vi "GraphSetup.vi"(8 "error in":errorcluster caption="entrée d'erreur (pas d'erreur)", 9 "AllowDef":bool, 10 "DataFileName":path, 11 "InterfaceIn":refnum<class "Interface.lvclass">) -> (0 "error out":errorcluster caption="sortie d'erreur", 3 "InterfaceOut":refnum<class "Interface.lvclass">)   [LabVIEW 2019, in "Interface.lvclass"]
uses:
  Interface.lvclass
  GraphSetupStates.ctl
  Interface.lvclass/Interface.ctl
  <vilib>/Utility/error.llb/DialogType.ctl
panel:
  out "DataIndex":i32[](array[numeric])
  out "DataCount":i32
  out "ScanlistItem":string
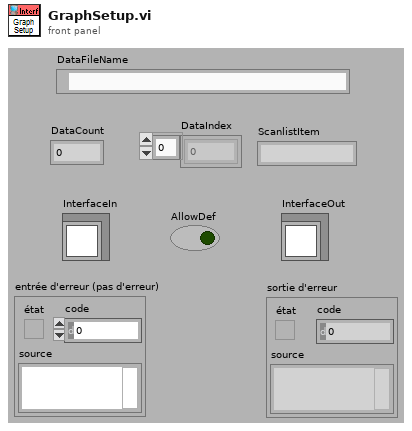
[diagram p1: front panel]
types:
  T1 = typedef "Interface.lvclass/GraphSetupStates.ctl" = enum16{"RdScnList", "UpdtGrphCurvs", "UpdtAllCurv", "SetGraphPar", "UpdtCrvPar", "GetNextItem", "UpdateGraph"}
  T2 = typedef "Interface.lvclass/CurveSetup.ctl" = cluster{"CurveName":string, "YParam":string, "XParam":string, "ZParam ":string, "GroupName":string, "LinWdth":u8, "PntCol":u32, "LinCol":u32, "LablFor":u8, "XScale":u32, "YScale":u32, "Interpol":u8, "DisplayName":string, "FillType":i16, "LineStyle":u8, "PntStyle":u8, "BarTyp":u8, "GraphIndex":i32, "Visible":bool, "XScaleName":string, "YScaleName":string, "XYGraph_Ref":refnum<vi>, "Data Only":bool, "DataQ Ref":refnum<queue>, "XParQ Ref":refnum<queue>, "XParamInd":i32, "ScanInd":i32, "File Path":path}
  T3 = typedef "DialogType.ctl" = u16
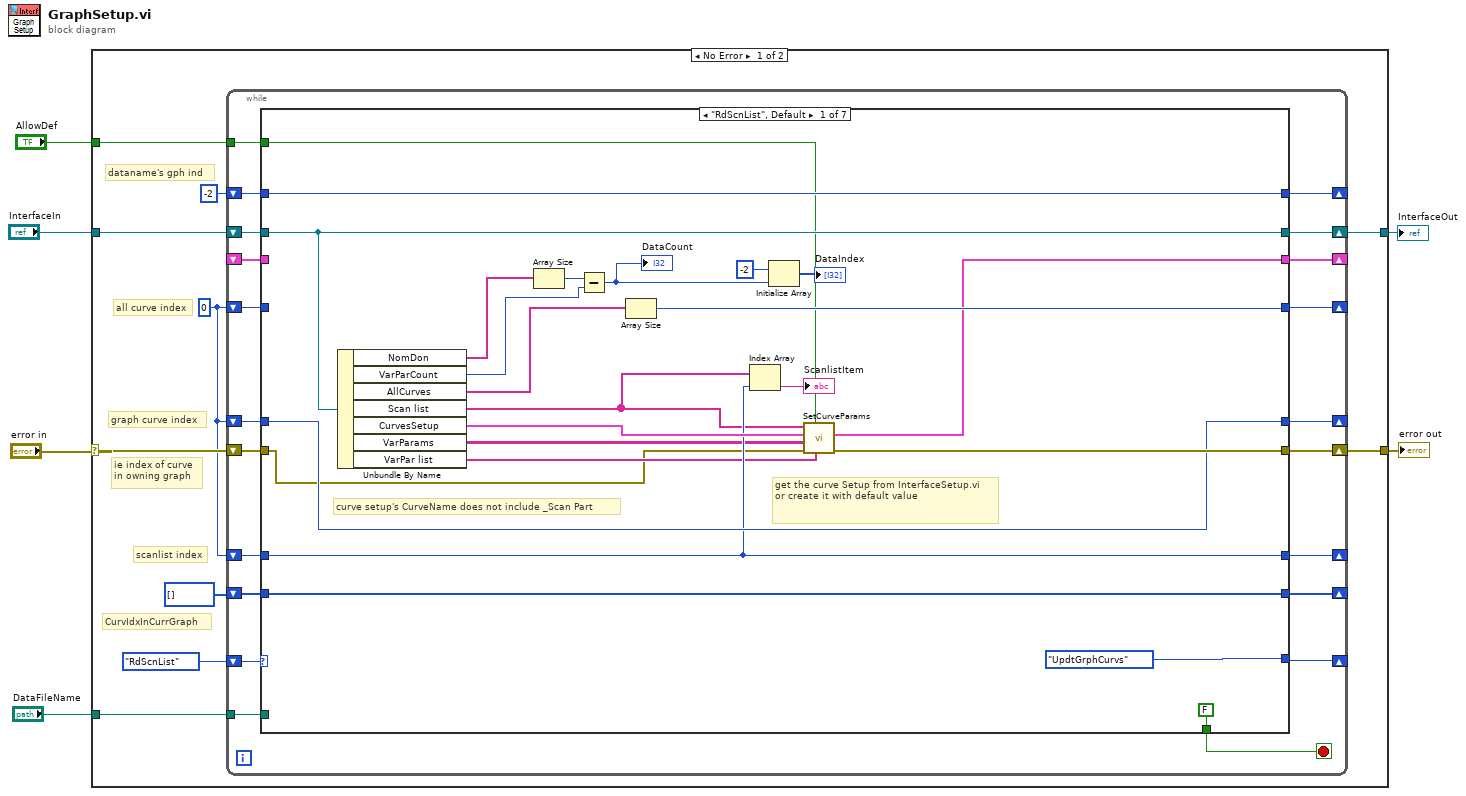
[diagram p0: block diagram]
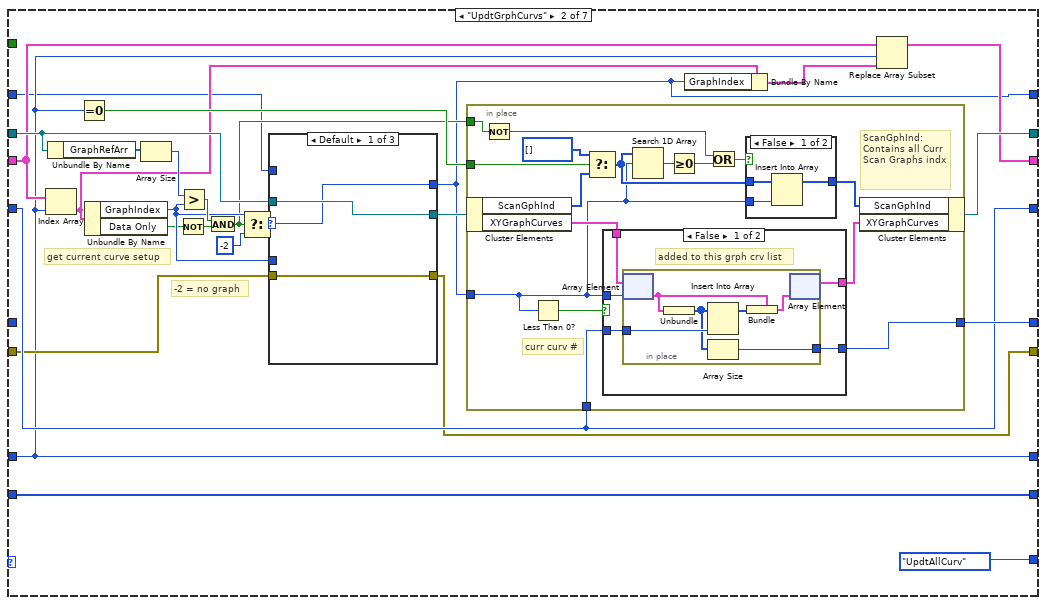
[diagram p2: hidden frame]
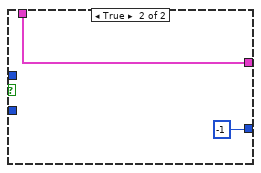
[diagram p3: hidden frame]
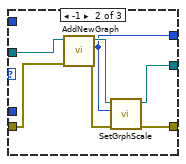
[diagram p5: hidden frame]
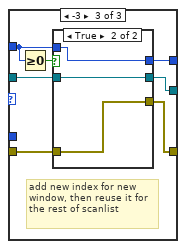
[diagram p6: hidden frame]
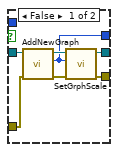
[diagram p7: hidden frame]
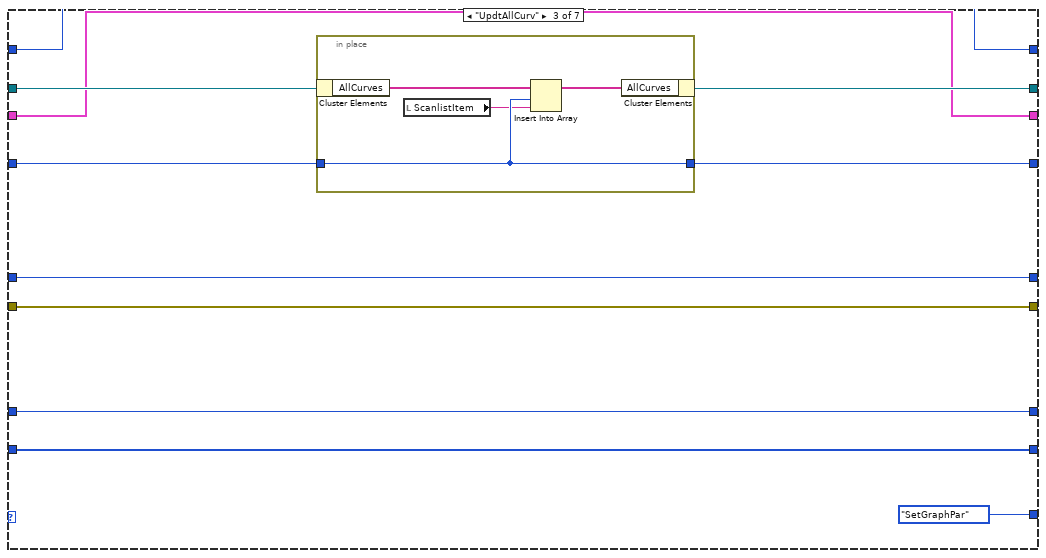
[diagram p8: hidden frame]
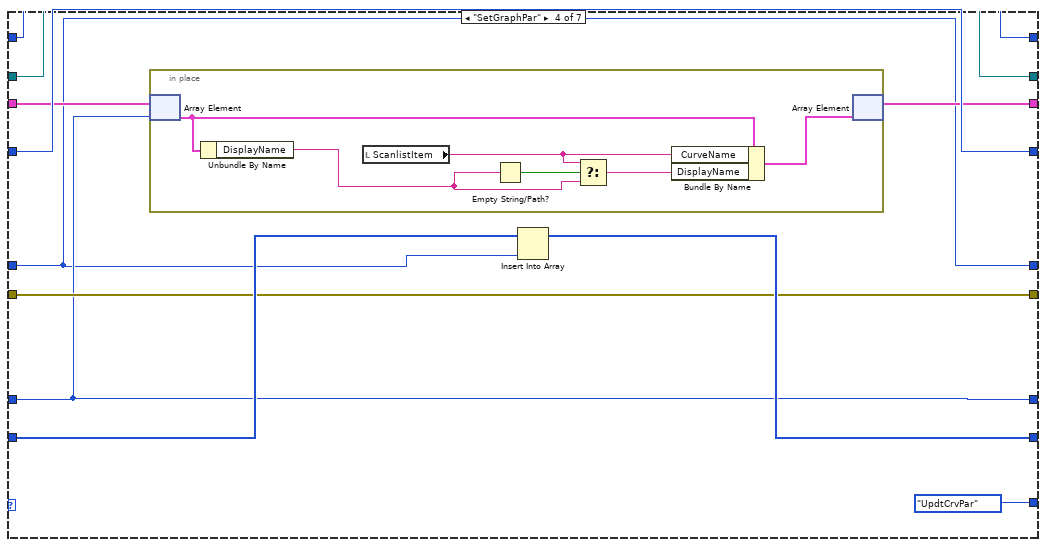
[diagram p9: hidden frame]
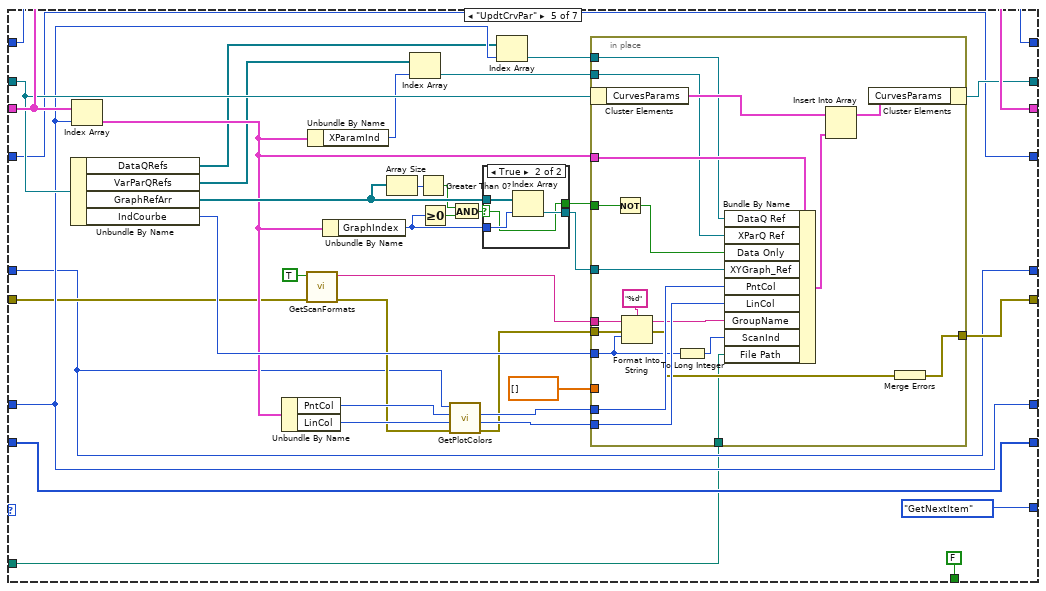
[diagram p10: hidden frame]
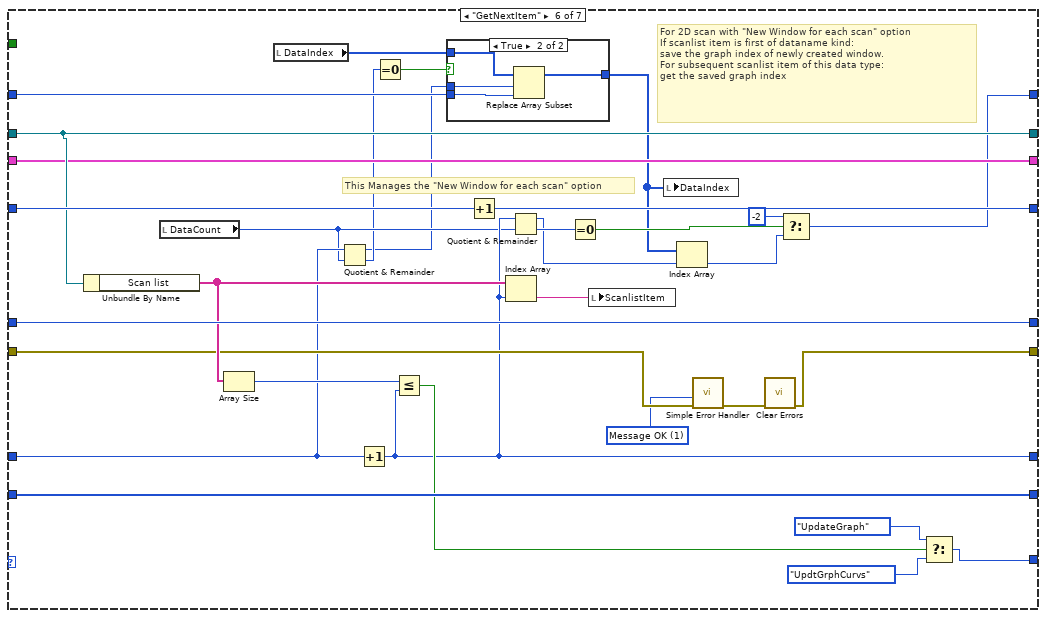
[diagram p12: hidden frame]
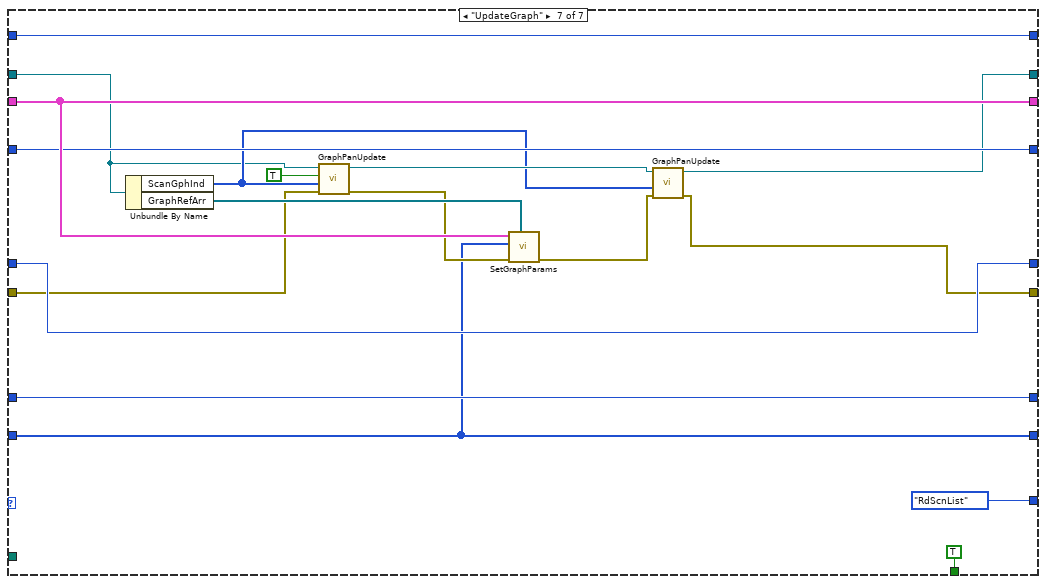
[diagram p14: hidden frame]
diagram:
  n1 = case shown="No Error" "error in" {
    selector: "error in" -> [w16 w298]
    tunnel: [w15 w298] -> w5
    tunnel: "InterfaceIn" -> [w12 w297]
    tunnel: [w13 w297] -> w3
    tunnel: "DataFileName" -> [w8 _]
    tunnel: "AllowDef" -> [w7 _]
    frame No Error {
      w10 = 0
      # "ie index of curve\nin owning graph"
      # "dataname's gph ind"
      # "CurvIdxInCurrGraph"
      # "scanlist index"
      # "graph curve index"
      # "all curve index"
      n2 = while {
        shift-right: [w28] -> w15
        shift-left: w16 -> [w29]
        shift-right: [w31] -> _
        shift-left: GraphSetupStates."RdScnList" ("Énum") -> [w23]
        shift-right: [w32] -> w13
        shift-left: w12 -> [w36]
        shift-right: [w35] -> _
        shift-left: w10 -> [w34]
        shift-right: [w33] -> _
        shift-left: w10 -> [w30]
        shift-right: [w27] -> _
        shift-left: _ -> [w26]
        shift-right: [w24] -> _
        shift-left: w10 -> [w25]
        shift-right: [w21] -> _
        shift-left: i32[] [] ("CuurGrphCrvInd") -> [w22]
        shift-right: [w20] -> _
        shift-left: -2 ("NewGraphInd") -> [w19]
        tunnel: w8 -> [w18]
        tunnel: w7 -> [w17]
        stop <- w37 stop-if-true
        n3 = case shown="\"RdScnList\", Default" w23 {
          tunnel: [FALSE _ _ _ FALSE _ TRUE] -> w37
          tunnel: w36 -> [w53 w80 w158 w171 w211 w270 w282]
          tunnel: [w59 w85 w154 w173 w190 w272 w290] -> w35
          tunnel: w34 -> [_ w85 w155 w173 w190 w273 w290]
          tunnel: [w54 w86 w150 w164 w181 w271 w294] -> w33
          tunnel: [w53 w81 w157 w171 w213 w270 w279] -> w32
          tunnel: [GraphSetupStates."UpdtGrphCurvs" ("Énum") GraphSetupStates."UpdtAllCurv" ("Énum") GraphSetupStates."SetGraphPar" ("Énum") GraphSetupStates."UpdtCrvPar" ("Énum") GraphSetupStates."GetNextItem" ("Énum") w257 GraphSetupStates."RdScnList" ("Énum")] -> w31
          tunnel: w30 -> [w54 _ w150 w164 w181 w271 w294]
          tunnel: w29 -> [w39 w84 w151 w168 w186 w264 w287]
          tunnel: [w56 w82 w151 w168 w205 w262 w280] -> w28
          tunnel: [w55 w71 w153 w166 w215 w269 w295] -> w27
          tunnel: w26 -> [_ w72 w153 w167 w215 w269 w295]
          tunnel: w25 -> [w50 w69 w152 w165 w191 w254 w293]
          tunnel: [w50 w69 w152 w165 w191 w256 w293] -> w24
          tunnel: w22 -> [w51 w64 w149 w170 w189 w261 w284]
          tunnel: [w51 w64 w149 w169 w189 w261 w284] -> w21
          tunnel: [w45 w63 w148 w163 w188 w246 w281] -> w20
          tunnel: w19 -> [w45 w62 w148 w163 w188 w255 w281]
          tunnel: w18 -> [_ _ _ _ w180 _ _]
          tunnel: w17 -> [w38 _ _ _ _ _ _]
          frame "RdScnList", Default {
            # "get the curve Setup from InterfaceSetup.vi\nor create it with default value"
            # "curve setup's CurveName does not include _Scan Part"
            n4 = Unbundle By Name(w53) -> ("NomDon"=w49:string[], "VarParCount"=w41:i32, "AllCurves"=w58:string[], "Scan list"=w40:string[], "CurvesSetup"=w61:T2[], "VarParams"=w44:string[][], "VarPar list"=w42:string[])
            n5 = Array Size(array=w49) -> (size(s)=w47:i32)
            n6 = Subtract(x=w47, y=w41) -> (x-y=w43:i32)
            "DataCount" <- w43
            n7 = Array Size(array=w58) -> (size(s)=w59:i32)
            n8 = Index Array(array=w40, index=w50) -> (element=→"ScanlistItem":string)
            n9 = Initialize Array(-2 ("NewGraphInd"), w43) -> (→"DataIndex":i32[])
            n10 = call "SetCurveParams.vi"("VarPar list"=w42, "AllowDef"=w38, "error in (no error)"=w39, "VarParams"=w44, "CurveSetupsIn"=w61, "CurveNames"=w40) -> ("error out"=w56:errorcluster, "CurveSetupsOut"=w55:T2[])  [unwired: 4 in]
          }
          frame "UpdtGrphCurvs" {
            # "-2 = no graph"
            # "get current curve setup"
            n11 = Index Array(array=w72, index=w69) -> (element=w70:T2)
            n12 = Unbundle By Name(w80) -> ("GraphRefArr"=w78:refnum<vi>[])
            n13 = Equal To 0?(x=w69) -> (x = 0?=w73:bool)
            n14 = Unbundle By Name(w70) -> ("GraphIndex"=w76:i32, "Data Only"=w67:bool)
            n15 = Array Size(array=w78) -> (size(s)=w79:i32)
            n16 = Not(x=w67) -> (.not. x?=w66:bool)
            n17 = Greater?(x=w79, y=w76) -> (0:w77:bool)
            n18 = And(x=w77, y=w66) -> (x .and. y?=w65:bool)
            n19 = Select(t=w76, s=w65, f=-2 ("cas faux")) -> (s? t:f=w74:i32)
            n20 = case shown="Default" w74 {
              selector: w74 -> [w121 _ _]
              tunnel: w76 -> [_ _ _]
              tunnel: [w121 w124 w133] -> w63
              tunnel: w80 -> [w123 w130 w137]
              tunnel: w84 -> [w122 w129 w136]
              tunnel: [w123 w127 w135] -> w83
              tunnel: [w122 w125 w134] -> w82
              tunnel: w62 -> [_ _ w131]
              frame Default {
              }
              frame -1 {
                n21 = call "AddNewGraph.vi"("error in (no error)"=w129, "Interface en entrée"=w130) -> ("error out"=w126:errorcluster, "NewGraphInd"=w124:i32, "Interface en sortie"=w128:refnum<class "Interface.lvclass">)  [unwired: 7 in]
                n22 = call "SetGrphScale.vi"("error in (no error)"=w126, "GraphIndex"=w124, "Interface en entrée"=w128) -> ("error out"=w125:errorcluster, "Interface en sortie"=w127:refnum<class "Interface.lvclass">)  [unwired: 7 in]
              }
              frame -3 {
                # "add new index for new window, then reuse it for the rest of scanlist"
                n23 = Greater Or Equal To 0?(x=w131) -> (x >= 0?=w132:bool)
                n24 = case shown="True" w132 {
                  tunnel: w137 -> [w144 w147]
                  tunnel: w136 -> [w143 w146]
                  tunnel: [w141 w147] -> w135
                  tunnel: [w139 w146] -> w134
                  tunnel: [w138 w145] -> w133
                  tunnel: w131 -> [_ w145]
                  frame False {
                    n25 = call "AddNewGraph.vi"("error in (no error)"=w143, "Interface en entrée"=w144) -> ("error out"=w140:errorcluster, "NewGraphInd"=w138:i32, "Interface en sortie"=w142:refnum<class "Interface.lvclass">)  [unwired: 7 in]
                    n26 = call "SetGrphScale.vi"("error in (no error)"=w140, "GraphIndex"=w138, "Interface en entrée"=w142) -> ("error out"=w139:errorcluster, "Interface en sortie"=w141:refnum<class "Interface.lvclass">)  [unwired: 7 in]
                  }
                  frame True {
                  }
                }
              }
            }
            n27 = in-place {
              in-place-border: [w103] -> w86
              in-place-border: w85 -> [w94]
              in-place-border: w73 -> [w102]
              in-place-border: w63 -> [w93]
              in-place-border: w65 -> [w90]
              # "curr curv #"
              # "ScanGphInd:\nContains all Curr Scan Graphs indx"
              n28 = in-place-cluster #1(w83) -> ("ScanGphInd"=w98:i32[], "XYGraphCurves"=w100:cluster{"Tableau":i32[]}[])
              n29 = Not(x=w90) -> (.not. x?=w89:bool)
              n30 = Less Than 0?(x=w93) -> (x < 0?=w92:bool)
              n31 = Select(t=i32[] [] ("cas vrai"), s=w102, f=w98) -> (s? t:f=w96:i32[])
              n32 = case shown="False" w92 {
                tunnel: [w108 -1] -> w103
                tunnel: w94 -> [w107 _]
                tunnel: w100 -> [w106 w116]
                tunnel: [w105 w116] -> w99
                tunnel: w93 -> [w104 _]
                frame False {
                  # "added to this grph crv list"
                  n33 = in-place {
                    in-place-border: [w114] -> w108
                    in-place-border: w107 -> [w113]
                    n34 = in-place-array #2(w106, w104) -> (w110:cluster{"Tableau":i32[]})
                    n35 = Unbundle(w110) -> ("Tableau"=w112:i32[])
                    n36 = Insert Into Array(array=w112, new element=w113) -> (w111:i32[])  [unwired: 1 in]
                    n37 = Array Size(array=w112) -> (size(s)=w114:i32)
                    n38 = Bundle(cluster=w110, "Tableau"=w111) -> (w109:cluster{"Tableau":i32[]})
                    n39 = in-place-array #2(w109) -> (w105:cluster{"Tableau":i32[]}[])  [unwired: 1 out]
                  }
                }
                frame True {
                }
              }
              n40 = Search 1D Array(1D array=w96, element=w93) -> (index of element=w95:i32)  [unwired: 1 in]
              n41 = Greater Or Equal To 0?(x=w95) -> (x >= 0?=w88:bool)
              n42 = Or(x=w89, y=w88) -> (x .or. y?=w91:bool)
              n43 = case shown="False" w91 {
                tunnel: [w119 w120] -> w97
                tunnel: w96 -> [w118 w120]
                tunnel: w93 -> [w117 _]
                frame False {
                  n44 = Insert Into Array(array=w118, new element=w117) -> (w119:i32[])  [unwired: 1 in]
                }
                frame True {
                  # "already in"
                }
              }
              n45 = in-place-cluster #1("ScanGphInd"=w97, "XYGraphCurves"=w99) -> (w81:refnum<class "Interface.lvclass">)
            }
            n46 = Bundle By Name(cluster=w70, "GraphIndex"=w63) -> (w68:T2)
            n47 = Replace Array Subset(array=w72, new element=w68, index=w69) -> (w71:T2[])
          }
          frame "UpdtAllCurv" {
            n48 = in-place {
              in-place-border: w155 -> [w160]
              in-place-border: [w160] -> w154
              n49 = in-place-cluster #3(w158) -> ("AllCurves"=w162:string[])
              n50 = local read "ScanlistItem"() -> (w159:string)
              n51 = Insert Into Array(array=w162, index=w160, new element=w159) -> (w161:string[])
              n52 = in-place-cluster #3("AllCurves"=w161) -> (w157:refnum<class "Interface.lvclass">)
            }
          }
          frame "SetGraphPar" {
            n53 = in-place {
              n54 = in-place-array #4(w167, w165) -> (w179:T2)
              n55 = Unbundle By Name(w179) -> ("DisplayName"=w177:string)
              n56 = local read "ScanlistItem"() -> (w176:string)
              n57 = Empty String/Path?(string/path=w177) -> (empty?=w178:bool)
              n58 = Select(t=w176, s=w178, f=w177) -> (s? t:f=w175:string)
              n59 = Bundle By Name(cluster=w179, "CurveName"=w176, "DisplayName"=w175) -> (w174:T2)
              n60 = in-place-array #4(w174) -> (w166:T2[])  [unwired: 1 out]
            }
            n61 = Insert Into Array(array=w170, new element=w164) -> (w169:i32[])  [unwired: 1 in]
          }
          frame "UpdtCrvPar" {
            n62 = Unbundle By Name(w211) -> ("DataQRefs"=w183:refnum<queue>[], "VarParQRefs"=w182:refnum<queue>[], "GraphRefArr"=w203:refnum<vi>[], "IndCourbe"=w206:i64)
            n63 = Index Array(array=w215, index=w191) -> (element=w195:T2)
            n64 = Unbundle By Name(w195) -> ("PntCol"=w210:u32, "LinCol"=w209:u32)
            n65 = call "GetScanFormats.vi"("ErrorIn(No Error)"=w186, "Scan(T)"=TRUE) -> ("sortie d'erreur"=w185:errorcluster, "Prefixe"=w187:string)  [unwired: 7 in, 1 out]
            n66 = Unbundle By Name(w195) -> ("XParamInd"=w194:i32)
            n67 = Unbundle By Name(w195) -> ("GraphIndex"=w204:i32)
            n68 = Array Size(array=w203) -> (size(s)=w199:i32)
            n69 = Index Array(array=w182, index=w194) -> (element=w193:refnum<queue>)
            n70 = Greater Than 0?(x=w199) -> (x > 0?=w200:bool)
            n71 = Greater Or Equal To 0?(x=w204) -> (x >= 0?=w201:bool)
            n72 = call "GetPlotColors.vi"("ErrorIn(No Error)"=w185, "Color2In"=w209, "Color1In"=w210, "ColorIndex"=w181) -> ("sortie d'erreur"=w192:errorcluster, "Color2Out"=w207:u32, "Color1Out"=w208:u32)  [unwired: 4 in, 1 out]
            n73 = And(x=w200, y=w201) -> (x .and. y?=w202:bool)
            n74 = case shown="True" w202 {
              selector: w202 -> [w217 w218]
              tunnel: [_ w221] -> w212
              tunnel: w203 -> [_ w220]
              tunnel: w204 -> [_ w219]
              tunnel: [w217 w218] -> w198
              frame False {
              }
              frame True {
                n75 = Index Array(array=w220, index=w219) -> (element=w221:refnum<vi>)
              }
            }
            n76 = Index Array(array=w183, index=w191) -> (element=w197:refnum<queue>)
            n77 = in-place {
              in-place-border: w212 -> [w239]
              in-place-border: w195 -> [w238]
              in-place-border: w208 -> [w236]
              in-place-border: w207 -> [w235]
              in-place-border: w187 -> [w233]
              in-place-border: w206 -> [w225]
              in-place-border: w192 -> [w228]
              in-place-border: [w227] -> w205
              in-place-border: w198 -> [w230]
              in-place-border: w197 -> [w223]
              in-place-border: dbl[] [] -> [_]
              in-place-border: w193 -> [w226]
              in-place-border: w180 -> [w222]
              n78 = in-place-cluster #5(w211) -> ("CurvesParams"=w241:T2[])
              n79 = Not(x=w230) -> (.not. x?=w229:bool)
              n80 = Format Into String(format string="%d" ("chaîne de format"), initial string=w233, error in=w228, w225) -> (resulting string=w232:string, error out=w231:errorcluster)
              n81 = To Long Integer(number=w225) -> (32bit integer=w224:i32)
              n82 = Bundle By Name(cluster=w238, "DataQ Ref"=w223, "XParQ Ref"=w226, "Data Only"=w229, "XYGraph_Ref"=w239, "PntCol"=w236, "LinCol"=w235, "GroupName"=w232, "ScanInd"=w224, "File Path"=w222) -> (w237:T2)
              n83 = Insert Into Array(array=w241, new element=w237) -> (w240:T2[])  [unwired: 1 in]
              n84 = in-place-cluster #5("CurvesParams"=w240) -> (w213:refnum<class "Interface.lvclass">)
              n85 = Merge Errors(w231) -> (w227:errorcluster)
            }
          }
          frame "GetNextItem" {
            w263 = T3 1 items=["pas de dialogue", "Message OK", "Message continuer ou arrêter", "Message OK + mises en garde", "Arrêter/Continuer + mises en garde"] ("type of dialog (OK msg:1)")
            # "For 2D scan with \"New Window for each scan\" option\nIf scanlist item is first of dataname kind:\nsave the graph index of newly created window.\nFor subsequent scanlist item of this data type:\nget the saved graph index"
            # "This Manages the \"New Window for each scan\" option"
            n86 = Unbundle By Name(w270) -> ("Scan list"=w267:string[])
            n87 = local read "DataCount"() -> (w253:i32)
            n88 = Array Size(array=w267) -> (size(s)=w268:i32)
            n89 = local read "DataIndex"() -> (w250:i32[])
            n90 = Quotient & Remainder(x=w254, y=w253) -> (x-y*floor(x/y)=w249:i32, floor(x/y)=w252:i32)
            n91 = Increment(x=w254) -> (x+1=w256:i32)
            n92 = Equal To 0?(x=w252) -> (x = 0?=w251:bool)
            n93 = Less Or Equal?(x=w268, y=w256) -> (x <= y?=w259:bool)
            n94 = case shown="True" w251 {
              tunnel: w255 -> [_ w277]
              tunnel: w250 -> [w274 w278]
              tunnel: w249 -> [_ w276]
              tunnel: [w274 w275] -> w245
              frame False {
              }
              frame True {
                n95 = Replace Array Subset(array=w278, new element=w277, index=w276) -> (w275:i32[])
              }
            }
            n96 = Increment(x=w273) -> (x+1=w272:i32)
            n97 = Index Array(array=w267, index=w256) -> (element=w266:string)
            n98 = Quotient & Remainder(x=w256, y=w253) -> (x-y*floor(x/y)=w244:i32, floor(x/y)=w247:i32)
            n99 = Equal To 0?(x=w247) -> (x = 0?=w248:bool)
            n100 = local write "ScanlistItem"(w266) -> ()
            n101 = local write "DataIndex"(w245) -> ()
            n102 = Index Array(array=w245, index=w244) -> (element=w243:i32)
            n103 = call <vilib>:"Simple Error Handler.vi"("type of dialog (OK msg:1)"=w263, "error in (no error)"=w264) -> ("error out"=w265:errorcluster)  [unwired: 3 in, 4 out]
            n104 = call <vilib>:"Clear Errors.vi"("error in (no error)"=w265) -> ("error out"=w262:errorcluster)  [unwired: 5 in, 1 out]
            n105 = Select(t=-2 ("cas vrai"), s=w248, f=w243) -> (s? t:f=w246:i32)
            n106 = Select(t=GraphSetupStates."UpdateGraph" ("Énum"), s=w259, f=GraphSetupStates."UpdtGrphCurvs" ("Énum")) -> (s? t:f=w257:T1)
          }
          frame "UpdateGraph" {
            n107 = Unbundle By Name(w282) -> ("ScanGphInd"=w283:i32[], "GraphRefArr"=w296:refnum<vi>[])
            n108 = call "GraphPanUpdate.vi"("error in (no error)"=w287, "GraphInd"=w283, "DeferUpdate"=TRUE, "Interface en entrée"=w282) -> ("error out"=w286:errorcluster, "Interface en sortie"=w288:refnum<class "Interface.lvclass">)  [unwired: 6 in]
            n109 = call "SetGraphParams.vi"("GraphRefArr"=w296, "error in"=w286, "CuurGrphCrvInd"=w284, "CurveSetupsIn"=w295) -> ("error out"=w285:errorcluster)  [unwired: 7 in]
            n110 = call "GraphPanUpdate.vi"("error in (no error)"=w285, "GraphInd"=w283, "Interface en entrée"=w288) -> ("error out"=w280:errorcluster, "Interface en sortie"=w279:refnum<class "Interface.lvclass">)  [unwired: 7 in]
          }
        }
      }
    }
    frame Error {
    }
  }
  "error out" <- w5
  "InterfaceOut" <- w3
